vi "read-json-testing.vi"() -> ()   [LabVIEW 2019]
uses:
  <vilib>/Rock Robotics/WPI/ThirdParty/MJansen/PathPlanner/TypeDef/PathPlannerPath.ctl
  <vilib>/Rock Robotics/WPI/ThirdParty/JAS_Junk/TrajLib/TypeDef/TRANSLATION2D.ctl
  <vilib>/Rock Robotics/WPI/ThirdParty/JAS_Junk/TrajLib/TypeDef/ROTATION2D.ctl
  <vilib>/Rock Robotics/WPI/ThirdParty/MJansen/PathPlanner/TypeDef/PathPlannerRotationTarget.ctl
  <vilib>/Rock Robotics/WPI/ThirdParty/MJansen/PathPlanner/TypeDef/PathPlannerConstraintsZone.ctl
  <vilib>/Rock Robotics/WPI/ThirdParty/MJansen/PathPlanner/TypeDef/PathPlannerPathConstraints.ctl
  <vilib>/Rock Robotics/WPI/ThirdParty/MJansen/PathPlanner/TypeDef/PathPlannerEventMarker.ctl
  <vilib>/Rock Robotics/WPI/ThirdParty/MJansen/PathPlanner/TypeDef/PathPlannerCommand.ctl
  <vilib>/Rock Robotics/WPI/ThirdParty/MJansen/PathPlanner/TypeDef/PathPlannerGoalEndState.ctl
  <vilib>/Rock Robotics/WPI/ThirdParty/MJansen/PathPlanner/TypeDef/PathPlannerPathPoint.ctl
  <vilib>/Rock Robotics/WPI/ThirdParty/MJansen/PathPlanner/TypeDef/PathPlannerTrajectory.ctl
  <vilib>/Rock Robotics/WPI/ThirdParty/MJansen/PathPlanner/TypeDef/PathPlannerTrajectoryState.ctl
  <vilib>/Rock Robotics/WPI/ThirdParty/JAS_Junk/TrajLib/TypeDef/CHASSIS_SPEEDS.ctl
  <vilib>/Rock Robotics/WPI/ThirdParty/MJansen/PathPlanner/PathPlanner24.lvlib
  <vilib>/Rock Robotics/WPI/ThirdParty/JAS_Junk/TrajLib/Trajectory_Library.lvlib
panel:
  in  "StartingSpeeds":T1 {"vOmega" format="%10.3f"; "vY" format="%10.3f"; "vX" format="%10.3f"}
  out "PathPlannerTrajectory":T2 {"States"."TargetHolonomicRotation"."SIN" format="%13.4f"; "States"."TargetHolonomicRotation"."COS" format="%13.4f"; "States"."TargetHolonomicRotation"."VALUE" format="%13.4f"; "States"."Heading"."SIN" format="%13.4f"; "States"."Heading"."COS" format="%13.4f"; "States"."Heading"."VALUE" format="%13.4f"; "States"."PositionMeters"."Y" format="%14.3f"; "States"."PositionMeters"."X" format="%14.3f"}
  out "Error":bool
  out "PathPlannerPath":T7={"BezierPoints"=[], "PreviewStartingRotation"={"VALUE"=0.0, "COS"=1.0, "SIN"=0.0}, "Reversed"=FALSE, "RotationTargets"=[], "ConstraintZones"=[], "EventMarkers"=[], "GlobalConstraints"={"MaxVelocityMps;"=0.0, "MaxAccelerationMpsSq;"=0.0, "MaxAngularVelRadPsEc;"=0.0, "MaxAngularAccRadPSecSq"=0.0, "Exists"=FALSE}, "GoalEndState"={"Velocity"=0.0, "Rotation"={"VALUE"=0.0, "COS"=1.0, "SIN"=0.0}}, "AllPoints"=[]} {"AllPoints"."HolonomicRotation"."SIN" format="%13.4f"; "AllPoints"."HolonomicRotation"."COS" format="%13.4f"; "AllPoints"."HolonomicRotation"."VALUE" format="%13.4f"; "AllPoints"."Position"."Y" format="%14.3f"; "AllPoints"."Position"."X" format="%14.3f"; "GoalEndState"."Rotation"."SIN" format="%13.4f"; "GoalEndState"."Rotation"."COS" format="%13.4f"; "GoalEndState"."Rotation"."VALUE" format="%13.4f"; "EventMarkers"."lastRobotPos"."Y" format="%14.3f"; "EventMarkers"."lastRobotPos"."X" format="%14.3f"; "EventMarkers"."markerPos"."Y" format="%14.3f"; "EventMarkers"."markerPos"."X" format="%14.3f"; "RotationTargets"."target"."SIN" format="%13.4f"; "RotationTargets"."target"."COS" format="%13.4f"; "RotationTargets"."target"."VALUE" format="%13.4f"; "PreviewStartingRotation"."SIN" format="%13.4f"; "PreviewStartingRotation"."COS" format="%13.4f"; "PreviewStartingRotation"."VALUE" format="%13.4f"; "BezierPoints"."Y" format="%14.3f"; "BezierPoints"."X" format="%14.3f"}
  out "value 7":T14(array[cluster])
  out "error out 7":errorcluster
  in  "path 7":string[](array[string])=["rotationTargets"]
  in  "rotationTargets":T14(array[cluster])
  out "value 6":T15(array[cluster])
  out "error out 6":errorcluster
  in  "path 6":string[](array[string])=["eventMarkers"]
  in  "eventMarkers":T15(array[cluster])
  out "value 5":T16(array[cluster])
  out "error out 5":errorcluster
  in  "path 5":string[](array[string])=["constraintZones"]
  in  "constraintZones":T16(array[cluster])
  out "value 4":cluster{"velocity":dbl, "rotation":dbl}
  in  "goalEndstate":cluster{"velocity":dbl, "rotation":dbl}
  out "error out 4":errorcluster
  in  "path 4":string[](array[string])=["goalEndState"]
  out "value 3":bool
  out "error out 3":errorcluster
  in  "path 3":string[](array[string])=["reversed"]
  in  "reversed":bool
  out "value 2":T17
  out "error out 2":errorcluster
  in  "path 2":string[](array[string])=["globalConstraints"]
  in  "globalConstraints":T17
  out "value":T18(array[cluster])
  in  "waypoints":T18(array[cluster])
  in  "enable LabVIEW extensions? (T)":bool=TRUE
  in  "strict validation? (F)":bool
  in  "default null elements? (F)":bool=TRUE
  out "error out":errorcluster
  in  "path":string[](array[string])=["waypoints"]
  in  "json source":string="{\n  \"version\": 1.0,\n  \"waypoints\": [\n    {\n      \"anchor\": {\n        \"x\": 2.0,\n        \"y\": 7.0\n      },\n      \"prevControl\": null,\n      \"nextControl\": {\n        \"x\": 3.575020864327443,\n        \"y\": 6.770873398889655\n      },\n      \"isLocked\": false\n    },\n    {\n      \"anchor\": {\n        \"x\": 5.951268188250662,\n        \"y\": 5.597064479843246\n      },\n      \"prevControl\": {\n        \"x\": 4.95424762677763,\n        \"y\": 6.594085041316277\n      },\n      \"nextControl\": {\n        \"x\": 6.951268188250662,\n        \"y\": 4.597064479843246\n      },\n      \"isLocked\": false\n    },\n    {\n      \"anchor\": {\n        \"x\": 7.0,\n        \"y\": 1.0\n      },\n      \"prevControl\": {\n        \"x\": 6.75,\n        \"y\": 2.5\n      },\n      \"nextControl\": null,\n      \"isLocked\": false\n    }\n  ],\n  \"rotationTargets\": [\n    {\n      \"waypointRelativePos\": 0.5,\n      \"rotationDegrees\": 0.0\n    }\n  ],\n  \"constraintZones\": [\n    {\n      \"name\": \"New Constraints Zone\",\n      \"minWaypointRelativePos\": 0.45,\n      \"maxWaypointRelativePos\": 0.7,\n      \"constraints\": {\n        \"maxVelocity\": 2.1,\n        \"maxAcceleration\": 2.2,\n        \"maxAngularVelocity\": 90.0,\n        \"maxAngularAcceleration\": 91.0\n      }\n    }\n  ],\n  \"eventMarkers\": [\n    {\n      \"name\": \"event-1\",\n      \"waypointRelativePos\": 0.6,\n      \"command\": {\n        \"type\": \"parallel\",\n        \"data\": {\n          \"commands\": [\n            {\n              \"type\": \"named\",\n              \"data\": {\n                \"name\": \"jim1\"\n              }\n            },\n            {\n              \"type\": \"named\",\n              \"data\": {\n                \"name\": \"jim2\"\n              }\n            }\n          ]\n        }\n      }\n    },\n    {\n      \"name\": \"event-2\",\n      \"waypointRelativePos\": 1.45,\n      \"command\": {\n        \"type\": \"sequential\",\n        \"data\": {\n          \"commands\": [\n            {\n              \"type\": \"named\",\n              \"data\": {\n                \"name\": \"jim3\"\n              }\n            }\n          ]\n        }\n      }\n    }\n  ],\n  \"globalConstraints\": {\n    \"maxVelocity\": 3,\n    \"maxAcceleration\": 3,\n    \"maxAngularVelocity\": 130.0,\n    \"maxAngularAcceleration\": 260.0\n  },\n  \"goalEndState\": {\n    \"velocity\": 0.0,\n    \"rotation\": -75.0\n  },\n  \"reversed\": false,\n  \"folder\": null,\n  \"previewStartingState\": null\n}"
  # "\"rotationTargets\": [\n    {\n      \"waypointRelativePos\": 0.5,\n      \"rotationDegrees\": 0.0\n    }\n  ],"
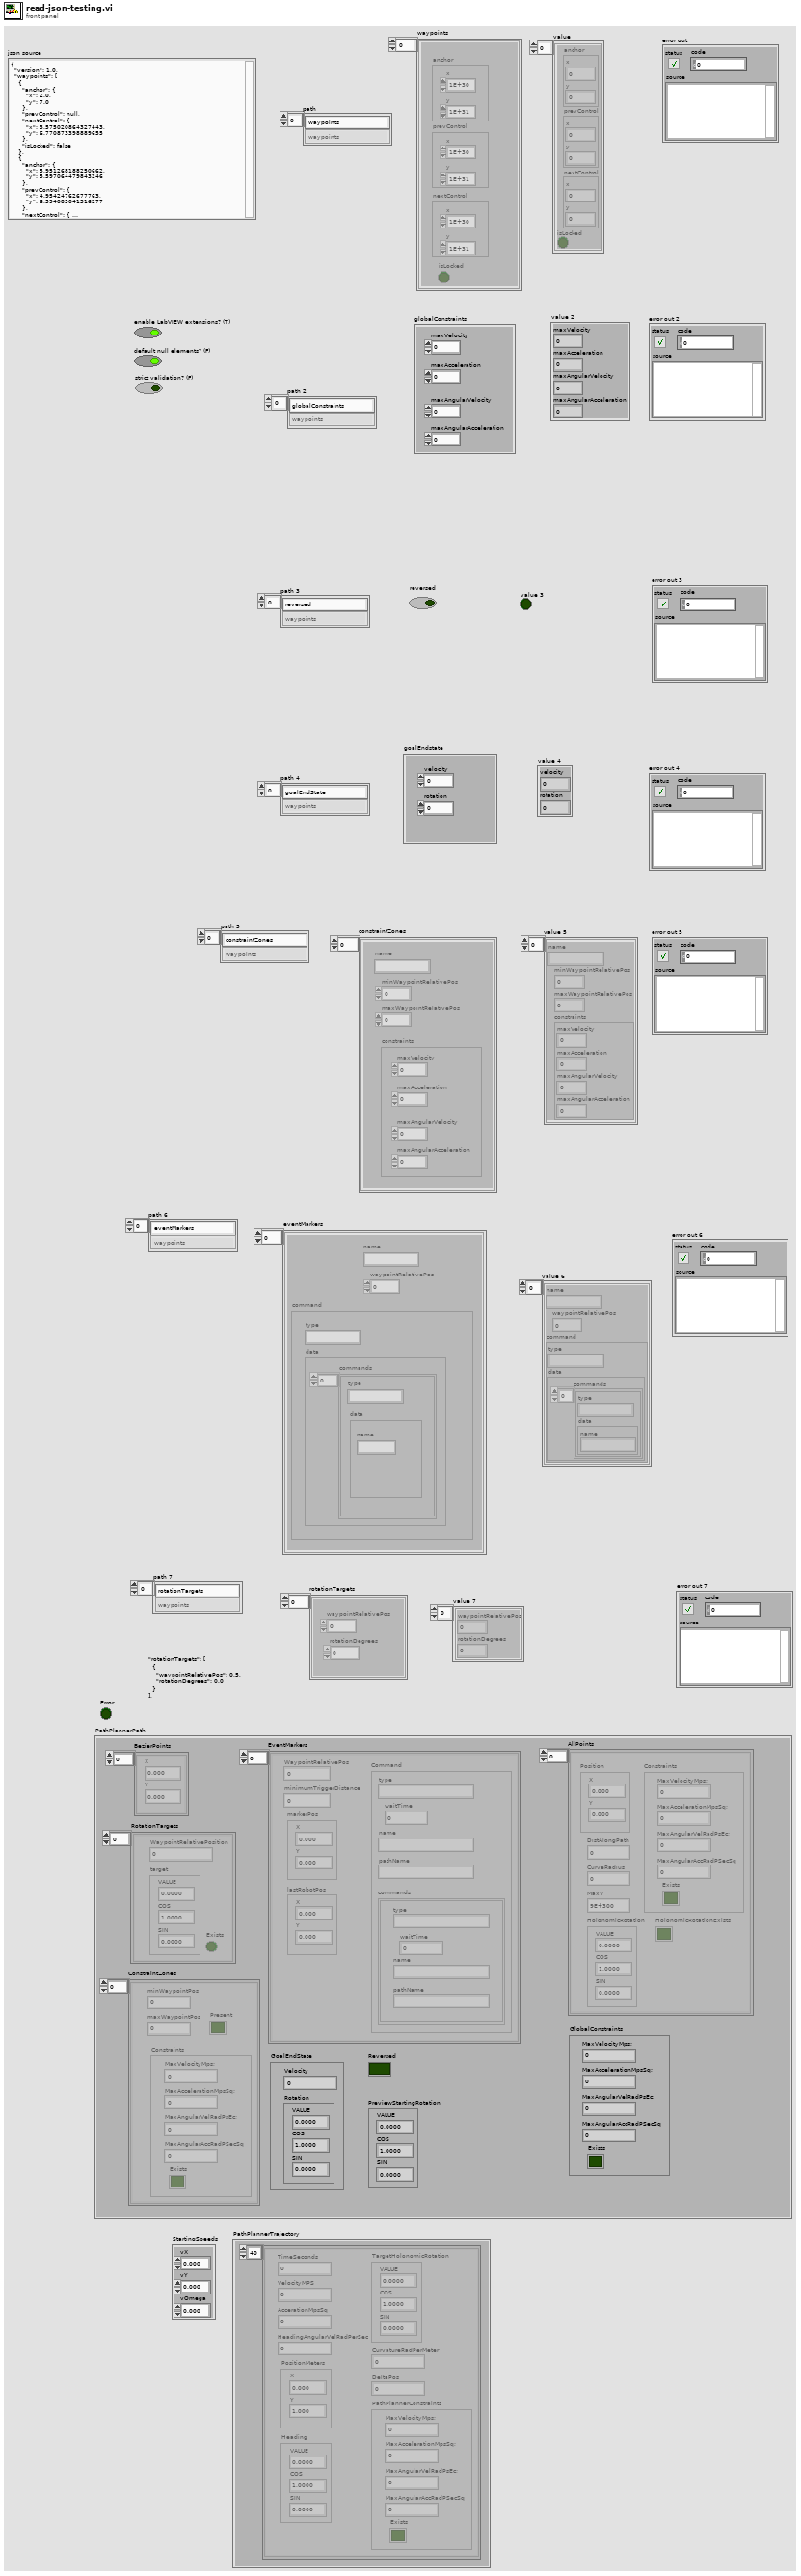
[diagram p1: front panel]
types:
  T1 = typedef "Trajectory_Library.lvlib/CHASSIS_SPEEDS.ctl" = cluster{"vX":dbl, "vY":dbl, "vOmega":dbl}
  T2 = typedef "PathPlanner24.lvlib/PathPlannerTrajectory.ctl" = cluster{"States":T3[]}
  T3 = typedef "PathPlanner24.lvlib/PathPlannerTrajectoryState.ctl" = cluster{"TimeSeconds":dbl, "VelocityMPS":dbl, "AccerationMpsSq":dbl, "HeadingAngularVelRadPerSec":dbl, "PositionMeters":T4, "Heading":T5, "TargetHolonomicRotation":T5, "CurvatureRadPerMeter":dbl, "PathPlannerConstraints":T6, "DeltaPos":dbl}
  T4 = typedef "Trajectory_Library.lvlib/TRANSLATION2D.ctl" = cluster{"X":dbl, "Y":dbl}
  T5 = typedef "Trajectory_Library.lvlib/ROTATION2D.ctl" = cluster{"VALUE":dbl, "COS":dbl, "SIN":dbl}
  T6 = typedef "PathPlanner24.lvlib/PathPlannerPathConstraints.ctl" = cluster{"MaxVelocityMps;":dbl, "MaxAccelerationMpsSq;":dbl, "MaxAngularVelRadPsEc;":dbl, "MaxAngularAccRadPSecSq":dbl, "Exists":bool}
  T7 = typedef "PathPlanner24.lvlib/PathPlannerPath.ctl" = cluster{"BezierPoints":T4[], "PreviewStartingRotation":T5, "Reversed":bool, "RotationTargets":T8[], "ConstraintZones":T9[], "EventMarkers":T10[], "GlobalConstraints":T6, "GoalEndState":T12, "AllPoints":T13[]}
  T8 = typedef "PathPlanner24.lvlib/PathPlannerRotationTarget.ctl" = cluster{"target":T5, "WaypointRelativePosition":dbl, "Exists":bool}
  T9 = typedef "PathPlanner24.lvlib/PathPlannerConstraintsZone.ctl" = cluster{"minWaypointPos":dbl, "maxWaypointPos":dbl, "Constraints":T6, "Present":bool}
  T10 = typedef "PathPlanner24.lvlib/PathPlannerEventMarker.ctl" = cluster{"WaypointRelativePos":dbl, "minimumTriggerDistance":dbl, "markerPos":T4, "lastRobotPos":T4, "Command":T11}
  T11 = typedef "PathPlanner24.lvlib/PathPlannerCommand.ctl" = cluster{"waitTime":dbl, "name":string, "type":string, "pathName":string, "commands":cluster{"type":string, "waitTime":dbl, "name":string, "pathName":string}[]}
  T12 = typedef "PathPlanner24.lvlib/PathPlannerGoalEndState.ctl" = cluster{"Velocity":dbl, "Rotation":T5}
  T13 = typedef "PathPlanner24.lvlib/PathPlannerPathPoint.ctl" = cluster{"Position":T4, "HolonomicRotation":T5, "DistAlongPath":dbl, "CurveRadius":dbl, "MaxV":dbl, "Constraints":T6, "HolonomicRotationExists":bool}
  T14 = cluster{"waypointRelativePos":dbl, "rotationDegrees":dbl}[]
  T15 = cluster{"name":string, "waypointRelativePos":dbl, "command":cluster{"type":string, "data":cluster{"commands":cluster{"type":string, "data":cluster{"name":string}}[]}}}[]
  T16 = cluster{"name":string, "minWaypointRelativePos":dbl, "maxWaypointRelativePos":dbl, "constraints":cluster{"maxVelocity":dbl, "maxAcceleration":dbl, "maxAngularVelocity":dbl, "maxAngularAcceleration":dbl}}[]
  T17 = cluster{"maxVelocity":dbl, "maxAcceleration":dbl, "maxAngularVelocity":dbl, "maxAngularAcceleration":dbl}
  T18 = cluster{"anchor":cluster{"x":dbl, "y":dbl}, "prevControl":cluster{"x":dbl, "y":dbl}, "nextControl":cluster{"x":dbl, "y":dbl}, "isLocked":bool}[]
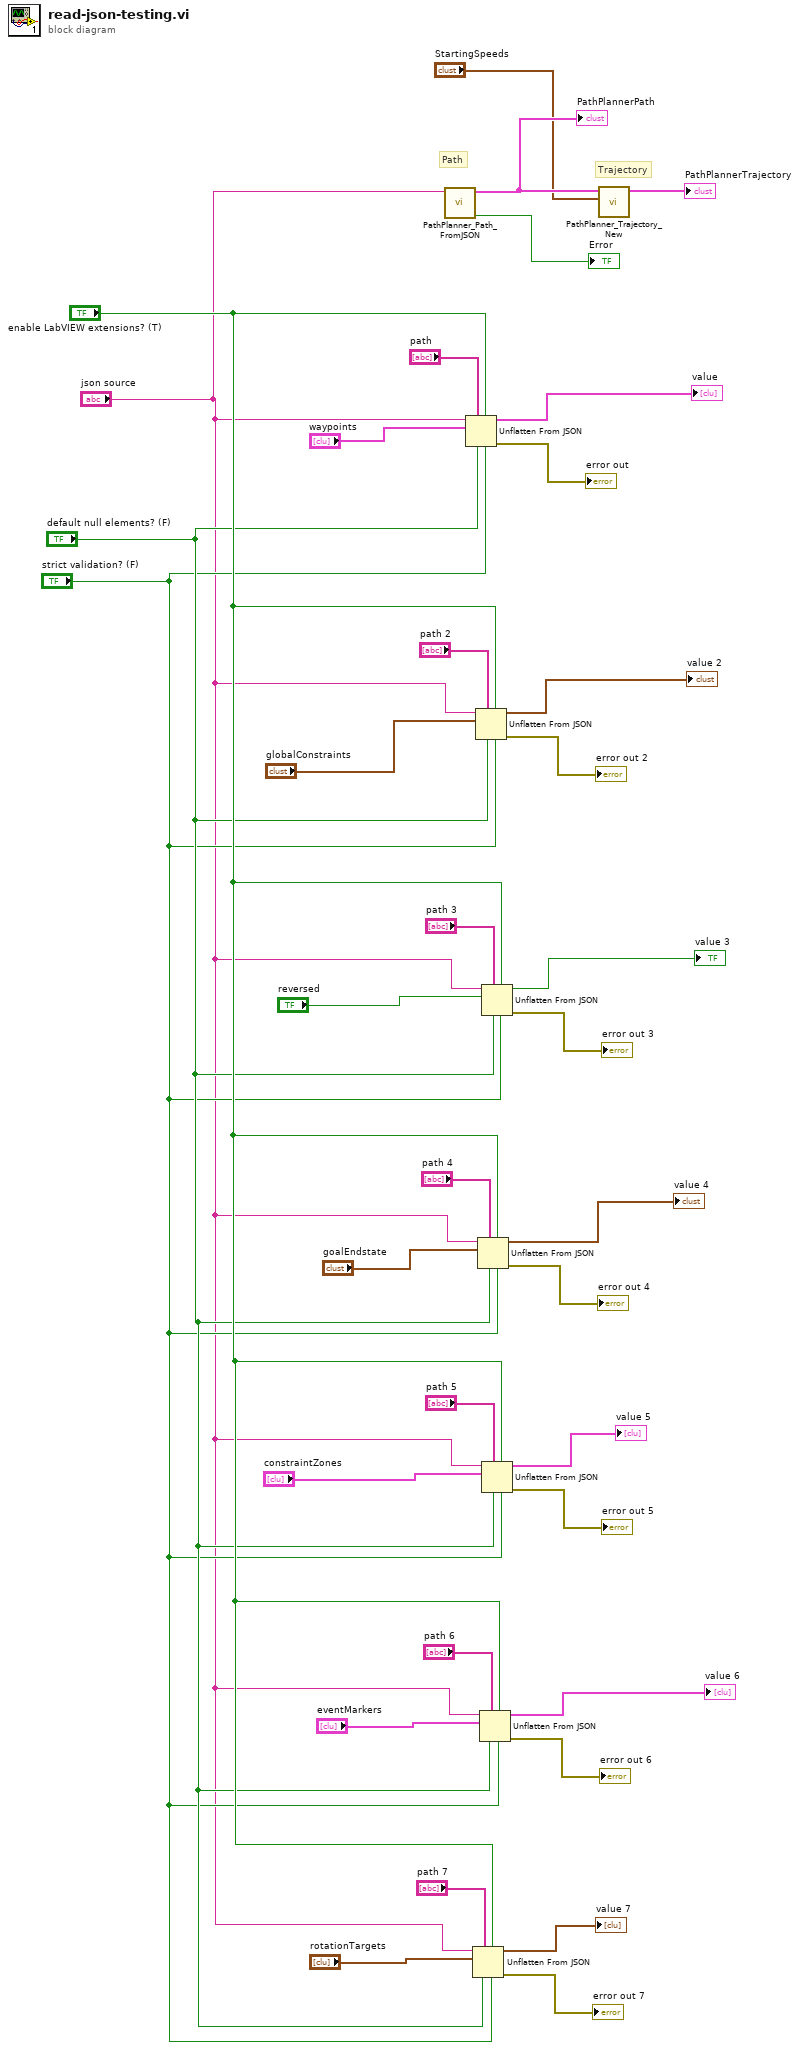
[diagram p0: block diagram]
diagram:
  # "Trajectory"
  # "Path"
  n1 = call <vilib>:"PathPlanner_Path_FromJSON.vi"("JSON String"="json source") -> ("Error"=→"Error":bool, "PathPlannerPath"=w3:T7)  [unwired: 9 in]
  "PathPlannerPath" <- w3
  n2 = Unflatten From JSON(path="path", enable LabVIEW extensions? (T)="enable LabVIEW extensions? (T)", JSON string="json source", type and defaults="waypoints", default null elements? (F)="default null elements? (F)", strict validation? (F)="strict validation? (F)") -> (value=→"value":T18, error out=→"error out":errorcluster)  [unwired: 1 in]
  n3 = Unflatten From JSON(path="path 7", enable LabVIEW extensions? (T)="enable LabVIEW extensions? (T)", JSON string="json source", type and defaults="rotationTargets", default null elements? (F)="default null elements? (F)", strict validation? (F)="strict validation? (F)") -> (value=→"value 7":T14, error out=→"error out 7":errorcluster)  [unwired: 1 in]
  n4 = Unflatten From JSON(path="path 2", enable LabVIEW extensions? (T)="enable LabVIEW extensions? (T)", JSON string="json source", type and defaults="globalConstraints", default null elements? (F)="default null elements? (F)", strict validation? (F)="strict validation? (F)") -> (value=→"value 2":T17, error out=→"error out 2":errorcluster)  [unwired: 1 in]
  n5 = Unflatten From JSON(path="path 4", enable LabVIEW extensions? (T)="enable LabVIEW extensions? (T)", JSON string="json source", type and defaults="goalEndstate", default null elements? (F)="default null elements? (F)", strict validation? (F)="strict validation? (F)") -> (value=→"value 4":cluster{"velocity":dbl, "rotation":dbl}, error out=→"error out 4":errorcluster)  [unwired: 1 in]
  n6 = Unflatten From JSON(path="path 6", enable LabVIEW extensions? (T)="enable LabVIEW extensions? (T)", JSON string="json source", type and defaults="eventMarkers", default null elements? (F)="default null elements? (F)", strict validation? (F)="strict validation? (F)") -> (value=→"value 6":T15, error out=→"error out 6":errorcluster)  [unwired: 1 in]
  n7 = Unflatten From JSON(path="path 3", enable LabVIEW extensions? (T)="enable LabVIEW extensions? (T)", JSON string="json source", type and defaults="reversed", default null elements? (F)="default null elements? (F)", strict validation? (F)="strict validation? (F)") -> (value=→"value 3":bool, error out=→"error out 3":errorcluster)  [unwired: 1 in]
  n8 = Unflatten From JSON(path="path 5", enable LabVIEW extensions? (T)="enable LabVIEW extensions? (T)", JSON string="json source", type and defaults="constraintZones", default null elements? (F)="default null elements? (F)", strict validation? (F)="strict validation? (F)") -> (value=→"value 5":T16, error out=→"error out 5":errorcluster)  [unwired: 1 in]
  n9 = call <vilib>:"PathPlanner_Trajectory_New.vi"("StartingSpeeds"="StartingSpeeds", "Path"=w3) -> ("PathPlannerTrajectory"=→"PathPlannerTrajectory":T2)  [unwired: 9 in]
